vi "Temperature.vi"() -> ()   [LabVIEW 2012]
doc: "Use this template to build a standard state machine design pattern. Each state executes code and determines which state to transition to. Contrast this design pattern with the User Interface Event Handler pattern, in which code executes in response to user actions. Contrast this design pattern also with the Queued Message Handler pattern, in which each message handling code can queue zero or more new messages.\nNote: This template does not contain the most recent programming guidelines recommended by National Instruments. For a complete, project-based implementation of the Standard State Machine pattern, use the Create Project dialog box instead of this template."
uses:
  temperatura.ctl
  <vilib>/DAQmx/write.llb/DAQmx Write (Analog DBL 1Chan 1Samp).vi
  <vilib>/DAQmx/read.llb/DAQmx Read (Analog 1D DBL 1Chan NSamp).vi
  <vilib>/DAQmx/create/channels.llb/DAQmx Create Channel (AI-Voltage-Basic).vi
  <vilib>/DAQmx/create/channels.llb/DAQmx Create Channel (AO-Voltage-Basic).vi
  <vilib>/DAQmx/miscellaneous.llb/DAQmx Fill In Error Info.vi
panel:
  in  "Slide":dbl(slide) min=0.0 max=5.0 scale=0.0..5.0
  in  "DAQmx Physical Channel 2":tag="Dev7/ai0"
  in  "stop":bool
  out "Waveform Chart":dbl(graph)
  in  "iloscOdczytow":dbl
  in  "DAQmx Physical Channel":tag="Dev7/ai0"
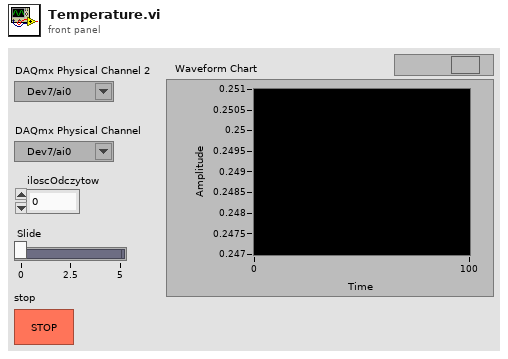
[diagram p1: front panel]
types:
  T1 = typedef "temperatura.ctl" = enum16{"Initialize", "Czytaj", "Grzej", "Stop", ""}
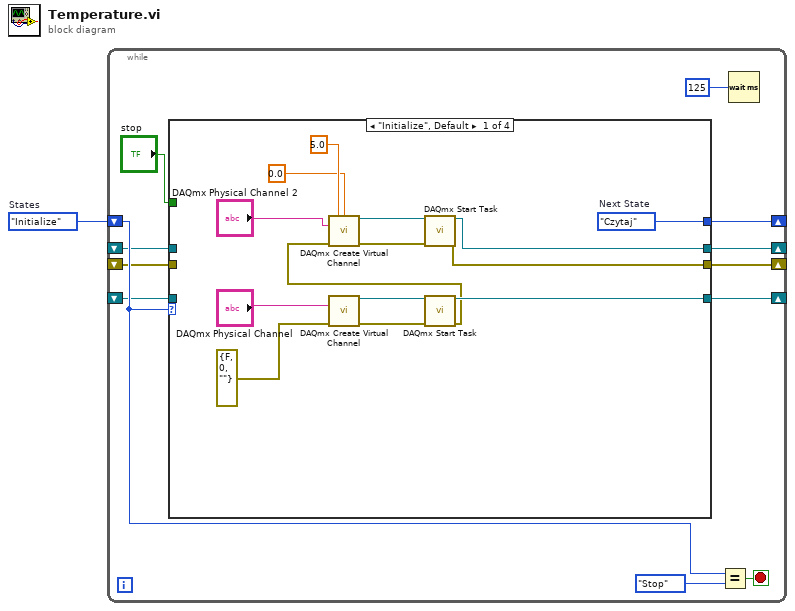
[diagram p0: block diagram]
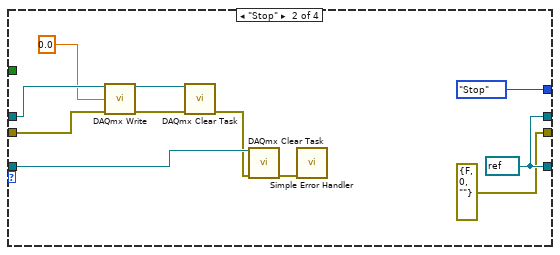
[diagram p2: hidden frame]
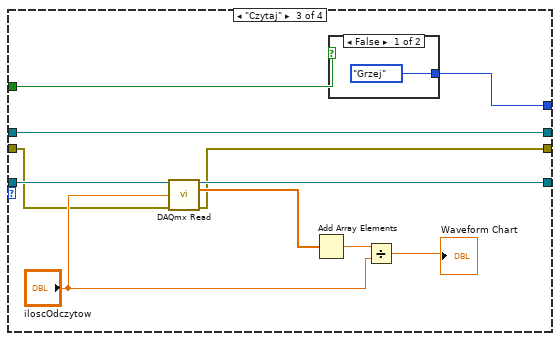
[diagram p3: hidden frame]
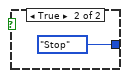
[diagram p4: hidden frame]
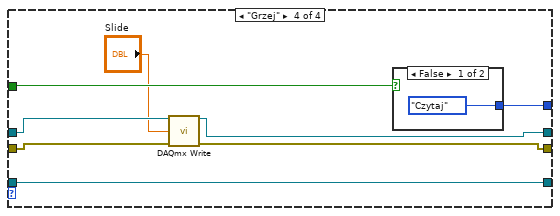
[diagram p5: hidden frame]
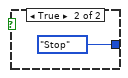
[diagram p6: hidden frame]
diagram:
  w1 = temperatura."Initialize"  # States
  n1 = while {
    shift-right: [w10] -> _
    shift-left: w1 -> [w11]
    shift-right: [w8] -> _
    shift-left: _ -> [w7]
    shift-right: [w5] -> _
    shift-left: _ -> [w3]
    shift-right: [w4] -> _
    shift-left: _ -> [w2]
    stop <- w13 stop-if-true
    n2 = case shown="\"Initialize\", Default" w11 {
      tunnel: [w27 temperatura."Stop" ("Next State") w43 w59] -> w10
      tunnel: [w23 w36 w48 w57] -> w8
      tunnel: w7 -> [_ w37 w49 w57]
      tunnel: "stop" -> [_ _ w42 w58]
      tunnel: [w20 w36 w41 w53] -> w5
      tunnel: [w18 errorcluster {"status"=FALSE, "code"=0, "source"=""} ("error out") w39 w52] -> w4
      tunnel: w3 -> [_ w34 w41 w56]
      tunnel: w2 -> [_ w33 w40 w55]
      frame "Initialize", Default {
        w27 = temperatura."Czytaj"  # Next State
        n3 = call-poly <vilib>:"DAQmx Create Virtual Channel.vi"("physical channels"="DAQmx Physical Channel", "error in"=errorcluster {"status"=FALSE, "code"=0, "source"=""}) -> ("task out"=w25:refnum<k21>, "error out"=w24:errorcluster)  [unwired: 12 in]
        n4 = call <vilib>:"DAQmx Start Task.vi"("task/channels in"=w25, "error in"=w24) -> ("task out"=w23:refnum<k21>, "error out"=w16:errorcluster)  [unwired: 12 in]
        n5 = call-poly <vilib>:"DAQmx Create Virtual Channel.vi"("maximum value"=5.0, "minimum value"=0.0, "physical channels"="DAQmx Physical Channel 2", "error in"=w16) -> ("task out"=w22:refnum<k21>, "error out"=w21:errorcluster)  [unwired: 10 in]
        n6 = call <vilib>:"DAQmx Start Task.vi"("task/channels in"=w22, "error in"=w21) -> ("task out"=w20:refnum<k21>, "error out"=w18:errorcluster)  [unwired: 12 in]
      }
      frame "Stop" {
        w36 = refnum<k21> refnum ("task out")
        n7 = call-poly <vilib>:"DAQmx Write.vi"("task/channels in"=w34, "data"=0.0, "error in"=w33) -> ("task out"=w32:refnum<k21>, "error out"=w31:errorcluster)  [unwired: 10 in, 1 out]
        n8 = call <vilib>:"DAQmx Clear Task.vi"("task in"=w32, "error in"=w31) -> ("error out"=w28:errorcluster)  [unwired: 13 in]
        n9 = call <vilib>:"DAQmx Clear Task.vi"("task in"=w37, "error in"=w28) -> ("error out"=w29:errorcluster)  [unwired: 13 in]
        n10 = call <vilib>:"Simple Error Handler.vi"("error in (no error)"=w29) -> ()  [unwired: 4 in, 5 out]
      }
      frame "Czytaj" {
        n11 = call-poly <vilib>:"DAQmx Read.vi"("task/channels in"=w49, "number of samples per channel"="iloscOdczytow", "error in"=w40) -> ("task out"=w48:refnum<k21>, "data"=w47:dbl[], "error out"=w39:errorcluster)  [unwired: 10 in]
        n12 = Add Array Elements(numeric array=w47) -> (sum=w46:dbl)
        n13 = case shown="False" w42 {
          tunnel: [temperatura."Grzej" ("Next State") temperatura."Stop" ("Next State")] -> w43
          frame False {
          }
          frame True {
          }
        }
        n14 = Divide(x=w46, y="iloscOdczytow") -> (x/y=→"Waveform Chart":dbl)
      }
      frame "Grzej" {
        n15 = call-poly <vilib>:"DAQmx Write.vi"("task/channels in"=w56, "data"="Slide", "error in"=w55) -> ("task out"=w53:refnum<k21>, "error out"=w52:errorcluster)  [unwired: 10 in, 1 out]
        n16 = case shown="False" w58 {
          tunnel: [temperatura."Czytaj" ("Next State") temperatura."Stop" ("Next State")] -> w59
          frame False {
          }
          frame True {
          }
        }
      }
    }
    n17 = Equal?(x=w11, y=temperatura."Stop" ("States")) -> (x = y?=w13:bool)
    n18 = Wait (ms)(milliseconds to wait=u32 125) -> ()  [unwired: 1 out]
  }
